vi "RPC.vi"(0 "mbed in":refnum<class "mbed.lvclass">, 5 "Name":string, 7 "method":string, 9 "Args":string[](array[string]), 11 "error in (no error)":errorcluster) -> (4 "mbed out":refnum<class "mbed.lvclass">, 8 "RPC Result":string, 15 "error out":errorcluster)   [LabVIEW 2011, in "mbed_LVLibrary.lvlib" / "mbed.lvclass"]
doc: "This VI is used to execute RPC commands on the mbed. It is a dynamic dispatch template and so calls the appropriate RPC VI from the transport classes depending on the constructor that was used."
uses:
  mbed.lvclass
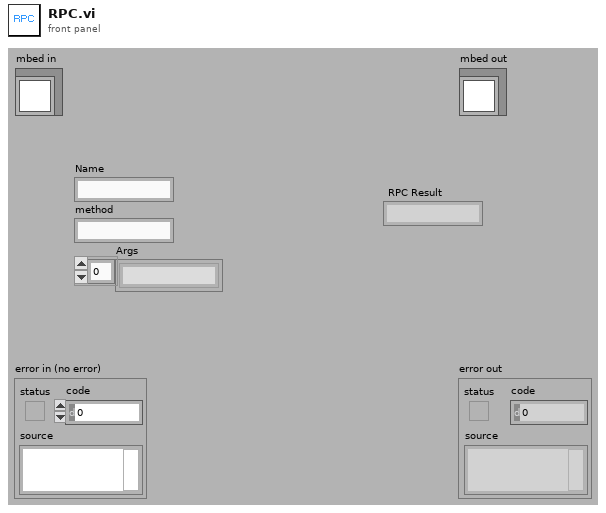
[diagram p1: front panel]
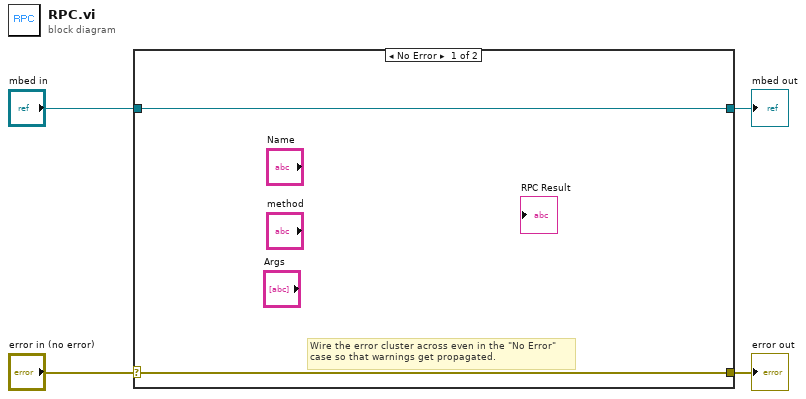
[diagram p0: block diagram]
diagram:
  n1 = case shown="No Error" "error in (no error)" {
    selector: "error in (no error)" -> [w5 w8]
    tunnel: [w5 w8] -> w3
    tunnel: [w6 w7] -> w1
    tunnel: "mbed in" -> [w6 w7]
    frame No Error {
      # "Wire the error cluster across even in the \"No Error\"\ncase so that warnings get propagated."
    }
    frame Error {
    }
  }
  "error out" <- w3
  "mbed out" <- w1
